vi "Waveform Edit.vi"(6 "Change in Time":i32, 9 "In Use Cluster":T1, 10 "New Data":dbl[][](array[numeric]), 11 "Old Data":dbl[][](array[numeric])) -> (1 "Overview Chart Data":waveform(dbl)[](array[waveform]), 2 "Output Waveform Cluster":T2, 3 "Output Decimated Data":dbl[][](array[numeric]))   [LabVIEW 2014]
panel:
  # "Waveform Edit VI"
  # "Inputs"
  # "Outputs"
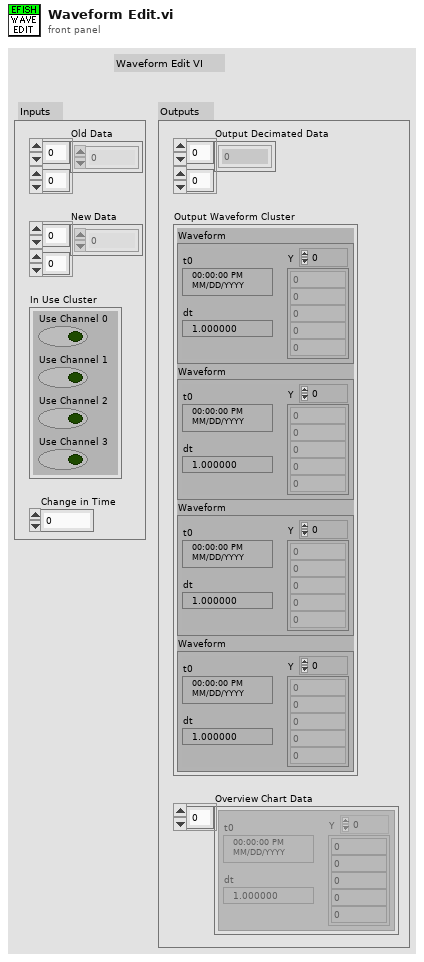
[diagram p1: front panel]
types:
  T1 = cluster{"Use Channel 0":bool, "Use Channel 1":bool, "Use Channel 2":bool, "Use Channel 3":bool}
  T2 = cluster{"Waveform":waveform(dbl), "Waveform":waveform(dbl), "Waveform":waveform(dbl), "Waveform":waveform(dbl)}
  T3 = cluster{"New Data":dbl[][], "Old Data":dbl[][], i32, i32, "Change in Time":i32, "Use Channel 1":bool}
  T4 = cluster{"New Data":dbl[][], "Old Data":dbl[][], i32, i32, "Change in Time":i32, "Use Channel 2":bool}
  T5 = cluster{"New Data":dbl[][], "Old Data":dbl[][], i32, i32, "Change in Time":i32, "Use Channel 3":bool}
  T6 = cluster{"New Data":dbl[][], "Old Data":dbl[][], i32, i32, "Change in Time":i32, "Use Channel 0":bool}
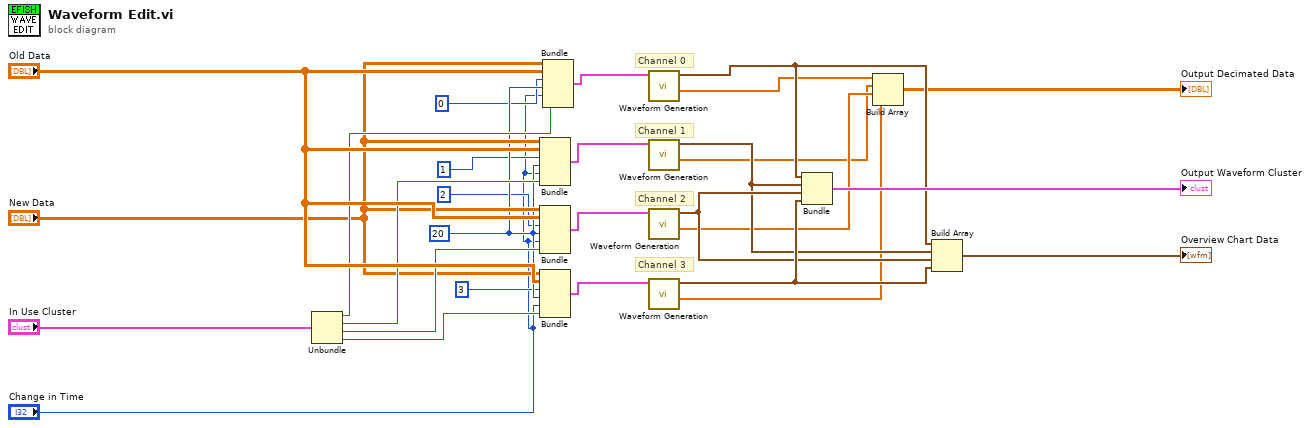
[diagram p0: block diagram]
diagram:
  w6 = 20
  # "Channel 3"
  # "Channel 2"
  # "Channel 1"
  # "Channel 0"
  n1 = Unbundle("In Use Cluster") -> ("Use Channel 0"=w9:bool, "Use Channel 1"=w10:bool, "Use Channel 2"=w11:bool, "Use Channel 3"=w12:bool)
  n2 = Bundle("New Data"="New Data", "Old Data"="Old Data", 1, w6, "Change in Time"="Change in Time", "Use Channel 1"=w10) -> (w15:T3)  [unwired: 1 in]
  n3 = Bundle("New Data"="New Data", "Old Data"="Old Data", 2, w6, "Change in Time"="Change in Time", "Use Channel 2"=w11) -> (w14:T4)  [unwired: 1 in]
  n4 = Bundle("New Data"="New Data", "Old Data"="Old Data", 3, w6, "Change in Time"="Change in Time", "Use Channel 3"=w12) -> (w13:T5)  [unwired: 1 in]
  n5 = Bundle("New Data"="New Data", "Old Data"="Old Data", 0, w6, "Change in Time"="Change in Time", "Use Channel 0"=w9) -> (w16:T6)  [unwired: 1 in]
  n6 = call "Waveform Generation.vi"("Cluster"=w16) -> ("Output Y Values"=w17:dbl[], "Waveform"=w24:waveform(dbl))  [unwired: 9 in]
  n7 = call "Waveform Generation.vi"("Cluster"=w15) -> ("Output Y Values"=w18:dbl[], "Waveform"=w25:waveform(dbl))  [unwired: 9 in]
  n8 = call "Waveform Generation.vi"("Cluster"=w14) -> ("Output Y Values"=w19:dbl[], "Waveform"=w26:waveform(dbl))  [unwired: 9 in]
  n9 = call "Waveform Generation.vi"("Cluster"=w13) -> ("Output Y Values"=w20:dbl[], "Waveform"=w27:waveform(dbl))  [unwired: 9 in]
  n10 = Bundle("Waveform"=w24, "Waveform"=w25, "Waveform"=w26, "Waveform"=w27) -> (→"Output Waveform Cluster":T2)  [unwired: 1 in]
  n11 = Build Array(w17, w18, w19, w20) -> (→"Output Decimated Data":dbl[][])
  n12 = Build Array(w24, w25, w26, w27) -> (→"Overview Chart Data":waveform(dbl)[])
